vi "read_excel.vi"(1 "file path (dialog if empty)":path caption="文件路径 （空时为对话框）") -> (0 "data_out":dbl[][](array[numeric]) format="%.6f")   [LabVIEW 2018]
uses:
  <vilib>/Utility/NIReport.llb/Report Type.ctl
  <vilib>/addons/_office/excel.llb/Excel Get Data ([str]).vi
  <vilib>/Utility/NIReport.llb/NI_report.lvclass
  <vilib>/Utility/NIReport.llb/NI_ReportGenerationCore.lvlib
  <vilib>/addons/_office/NI_ReportGenerationToolkit.lvlib
  <vilib>/Utility/NIReport.llb/Excel/NI_Excel.lvclass
panel:
  out "data":string[][](array[string])
  in  "error in (no error)":errorcluster caption="错误输入（无错误）"
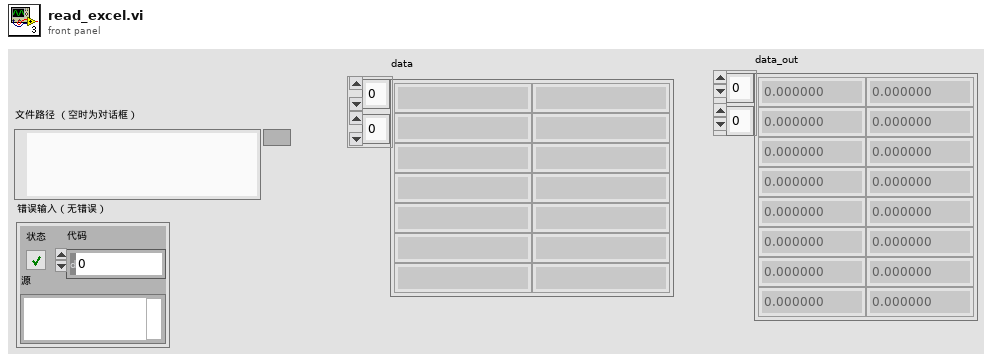
[diagram p1: front panel]
types:
  T1 = typedef "NI_ReportGenerationCore.lvlib/Report Type.ctl" = enum16{"HTML", "Word", "Excel"}
  T2 = enum16{"maximized", "minimized", "normal", "no change"}
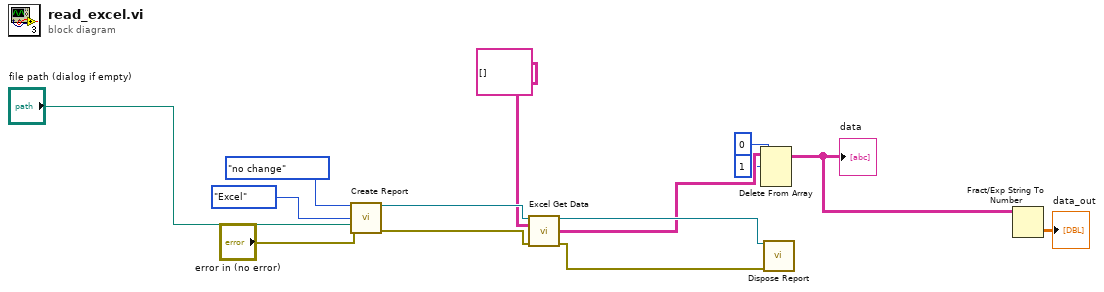
[diagram p0: block diagram]
diagram:
  n1 = call <vilib>:"Create Report.vi"("window state (normal)"=T2."no change", "report type"=Report_Type."Excel", "template (empty)"="file path (dialog if empty)", "error in (no error)"="error in (no error)") -> ("report out"=w11:refnum<class "NI_report.lvclass">, "error out"=w7:errorcluster)  [unwired: 10 in]
  n2 = call-poly <vilib>:"Excel Get Data.vi"("report in"=w11, "data type"=string[][] [], "error in (no error)"=w7) -> ("report out"=w9:refnum<class "NI_report.lvclass">, "data"=w5:string[][], "error out"=w8:errorcluster)  [unwired: 10 in]
  n3 = Delete From Array(array=w5, length=1 ("长度"), index (row)=0 ("索引 (行)")) -> (array with subset deleted=w2:string[][])  [unwired: 1 in, 1 out]
  "data" <- w2
  n4 = call-dynamic "Dispose Report.vi"("report in"=w9, "error in (no error)"=w8) -> ()  [unwired: 13 in, 1 out]
  n5 = Fract/Exp String To Number(string=w2) -> (number=→"data_out":dbl[][])  [unwired: 3 in, 1 out]
